vi "Get SMO HELP getAll.vi"(8 "error in (no error)":errorcluster, 11 "Instrument.AFM_DLog in":refnum<class "Instrument.AFM_DLog.lvclass">) -> (0 "error out":errorcluster, 2 "getall cluster":variant, 3 "Instrument.AFM_DLog out":refnum<class "Instrument.AFM_DLog.lvclass">)   [LabVIEW 2019, in "Instrument.AFM_DLog.lvclass"]
uses:
  Instrument.AFM_DLog.lvclass
  Typedefs/Instrument.AFM_DLog.getAll--Cluster.ctl
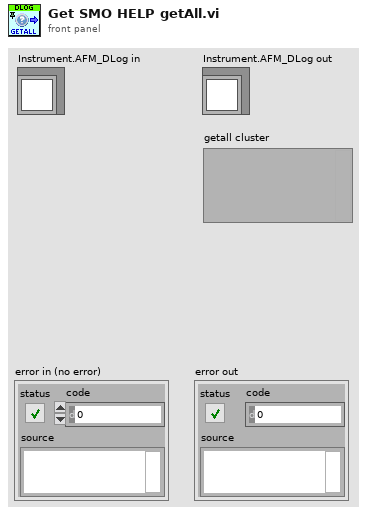
[diagram p1: front panel]
types:
  T1 = typedef "Instrument.AFM_DLog.lvclass/Instrument.AFM_DLog.getAll--Cluster.ctl" = cluster{"Name":string, "Time":string, "X":dbl, "Y":dbl, "Speed":dbl, "Voltage":dbl, "Set Resistance":string}
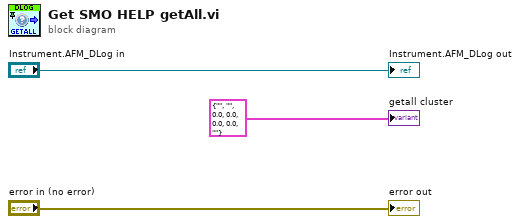
[diagram p0: block diagram]
diagram:
  "Instrument.AFM_DLog out" <- "Instrument.AFM_DLog in"
  "error out" <- "error in (no error)"
  "getall cluster" <- T1 {"Name"="", "Time"="", "X"=0.0, "Y"=0.0, "Speed"=0.0, "Voltage"=0.0, "Set Resistance"=""}
